vi "Created Send.vi"   [LabVIEW 2025]
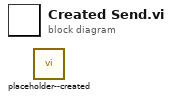
[diagram p0: block diagram]
diagram:
  n1 = call "placeholder--created.vi"() -> ()  [unwired: 11 in, 1 out]
